vi "CollectData.vi"(11 "read buffer":string) -> (0 "Static Load Force (LF)":dbl, 1 "Elbow Angle":dbl, 2 "Grip Force (GF)":dbl, 3 "Dynamic Load Force (LF)":dbl)   [LabVIEW 2018]
panel:
  # "Input"
  # "Outputs"
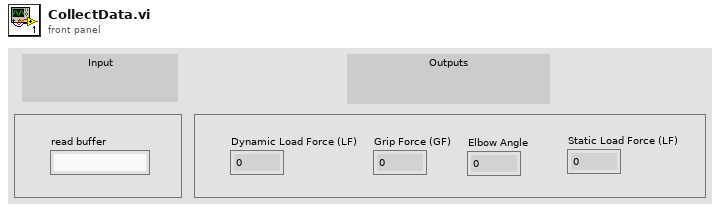
[diagram p1: front panel]
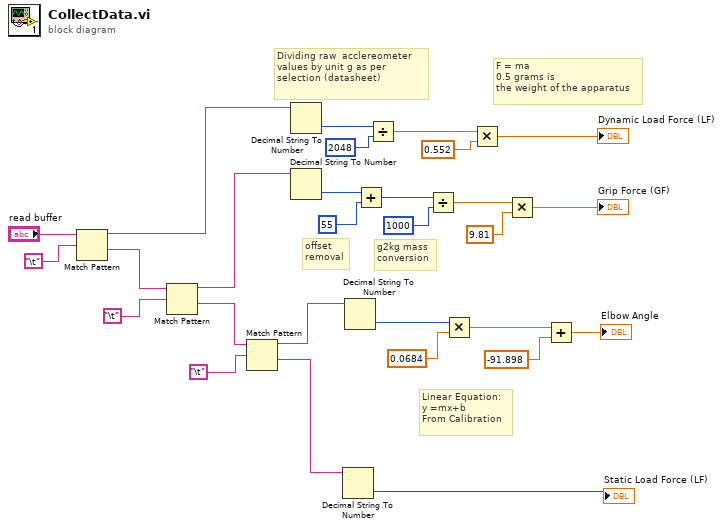
[diagram p0: block diagram]
diagram:
  # "Dividing raw  acclereometer\nvalues by unit g as per selection (datasheet)"
  # "F = ma\n0.5 grams is \nthe weight of the apparatus"
  # "g2kg mass\nconversion"
  # "offset\nremoval"
  # "Linear Equation:\ny =mx+b\nFrom Calibration"
  n1 = Match Pattern(string="read buffer", regular expression="\t") -> (before substring=w23:string, after substring=w12:string)  [unwired: 1 in, 2 out]
  n2 = Match Pattern(string=w12, regular expression="\t") -> (before substring=w11:string, after substring=w4:string)  [unwired: 1 in, 2 out]
  n3 = Match Pattern(string=w4, regular expression="\t") -> (before substring=w3:string, after substring=w2:string)  [unwired: 1 in, 2 out]
  n4 = Decimal String To Number(string=w23) -> (number=w17:i32)  [unwired: 2 in, 1 out]
  n5 = Decimal String To Number(string=w11) -> (number=w25:i32)  [unwired: 2 in, 1 out]
  n6 = Decimal String To Number(string=w2) -> (number=→"Static Load Force (LF)":i32)  [unwired: 2 in, 1 out]
  n7 = Decimal String To Number(string=w3) -> (number=w7:i32)  [unwired: 2 in, 1 out]
  n8 = Add(x=w25, y=55) -> (x+y=w27:i32)
  n9 = Divide(x=w17, y=2048) -> (x/y=w16:dbl)
  n10 = Divide(x=w27, y=1000) -> (x/y=w20:dbl)
  n11 = Multiply(x=w7, y=0.0684 ("x")) -> (x*y=w10:dbl)
  n12 = Multiply(x=w16, y=0.552) -> (x*y=→"Dynamic Load Force (LF)":dbl)
  n13 = Multiply(x=w20, y=9.81) -> (x*y=→"Grip Force (GF)":dbl)
  n14 = Add(x=w10, y=-91.898 ("x")) -> (x+y=→"Elbow Angle":dbl)
